vi "Set MenuItem Properties.vi"(0 "NotifyIcon in":refnum<class "NotifyIcon.lvclass">, 5 "MenuItem":refnum<k24>, 9 "MenuItem Properties":T1={"Enabled"=TRUE, "Visible"=TRUE, "DefaultItem"=FALSE, "Checked"=FALSE, "RadioCheck"=FALSE, "Break"=FALSE, "BarBreak"=FALSE, "Text"=""}, 11 "error in (no error)":errorcluster) -> (4 "dub NotifyIcon":refnum<class "NotifyIcon.lvclass">, 6 "MenuItem out":refnum<k24>, 15 "error out":errorcluster)   [LabVIEW 2016, in "NotifyIcon.lvclass"]
doc: "This VI sets the properties for the MenuItem referenced by the <b>MenuItem</b> input.\n\n\nStinus Olsen\nCIM Industrial Systems A/S\n22. Feb. 2011 15:06\nmailto: seo@cim.as"
uses:
  NotifyIcon.lvclass
  System.Windows.Forms
  Controls/MenuItem Properties.ctl
panel:
  # "This VI belongs to the NotifyIcon Toolset. \nA toolset that makes it easy to create, control and manipulate a notification icon in the notification area of the Windows taskbar.\nThe toolset requires Microsoft .NET framework 2.0\n\n\nNOTICE -- YOU MUST LEAVE THIS NOTICE IN PLACE.  PER THE TERMS OF THE LICENSE BELOW, YOU MAY SUBLICENSE THIS SOFTWARE \nIN ANY WAY THAT DOES NOT CONFLICT WITH THIS LICENSE.\n\n### BSD License (http://www.opensource.org/licenses/bsd-license.php) Begin ###\n \nCopyright (c) 2011, Stinus Olsen <seo@cim.as>\n\nAll rights reserved.\n\nRedistribution and use in source and binary forms, with or without modification, are permitted provided that the following conditions are met:\n\n    * Redistributions of source code must retain the above copyright notice, this list of conditions and the following disclaimer.\n    * Redistributions in binary form must reproduce the above copyright notice, this list of conditions and the following disclaimer in the \n       documentation and/or other materials provided with the distribution.\n    * Neither the name of CIM Industrial Systems nor the names of its contributors may be used to endorse or promote products derived \n       from this software without specific prior written permission.\n\nTHIS SOFTWARE IS PROVIDED BY THE COPYRIGHT HOLDERS AND CONTRIBUTORS \"AS IS\" AND ANY EXPRESS OR IMPLIED WARRANTIES, \nINCLUDING, BUT NOT LIMITED TO, THE IMPLIED WARRANTIES OF MERCHANTABILITY AND FITNESS FOR A PARTICULAR PURPOSE ARE \nDISCLAIMED. IN NO EVENT SHALL THE COPYRIGHT OWNER OR CONTRIBUTORS BE LIABLE FOR ANY DIRECT, INDIRECT, INCIDENTAL,\n SPECIAL, EXEMPLARY, OR CONSEQUENTIAL DAMAGES (INCLUDING, BUT NOT LIMITED TO, PROCUREMENT OF SUBSTITUTE GOODS OR \nSERVICES; LOSS OF USE, DATA, OR PROFITS; OR BUSINESS INTERRUPTION) HOWEVER CAUSED AND ON ANY THEORY OF LIABILITY, \nWHETHER IN CONTRACT, STRICT LIABILITY, OR TORT (INCLUDING NEGLIGENCE OR OTHERWISE) ARISING IN ANY WAY OUT OF THE USE \nOF THIS SOFTWARE, EVEN IF ADVISED OF THE POSSIBILITY OF SUCH DAMAGE.\n\n### BSD License End ###"
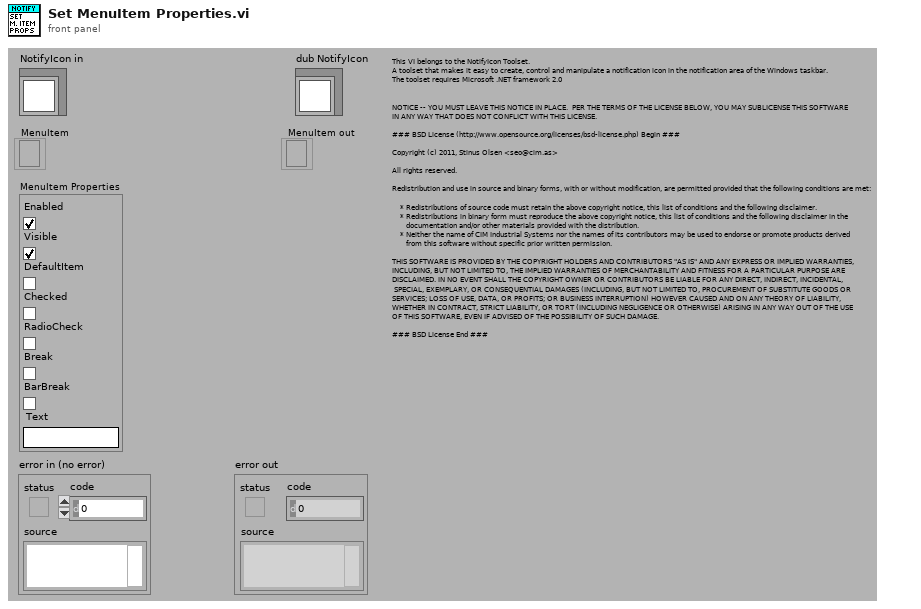
[diagram p1: front panel]
types:
  T1 = typedef "NotifyIcon.lvclass/MenuItem Properties.ctl" = cluster{"Enabled":bool, "Visible":bool, "DefaultItem":bool, "Checked":bool, "RadioCheck":bool, "Break":bool, "BarBreak":bool, "Text":string}
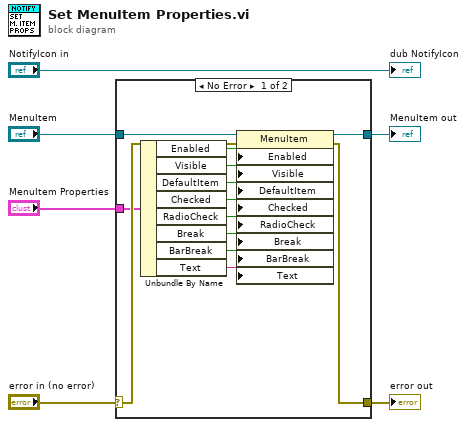
[diagram p0: block diagram]
diagram:
  n1 = case shown="No Error" "error in (no error)" {
    selector: "error in (no error)" -> [w18 w21]
    tunnel: [w17 w21] -> w5
    tunnel: "MenuItem" -> [w19 w20]
    tunnel: [w16 w20] -> w2
    tunnel: "MenuItem Properties" -> [w15 _]
    frame No Error {
      n2 = Unbundle By Name(w15) -> ("Enabled"=w14:bool, "Visible"=w13:bool, "DefaultItem"=w12:bool, "Checked"=w11:bool, "RadioCheck"=w10:bool, "Break"=w9:bool, "BarBreak"=w8:bool, "Text"=w7:string)
      n3 = property class="MenuItem"(reference=w19, error in=w18, "Enabled"=w14, "Visible"=w13, "DefaultItem"=w12, "Checked"=w11, "RadioCheck"=w10, "Break"=w9, "BarBreak"=w8, "Text"=w7) -> (reference out=w16:refnum<k24>, error out=w17:errorcluster)
    }
    frame Error {
    }
  }
  "error out" <- w5
  "MenuItem out" <- w2
  "dub NotifyIcon" <- "NotifyIcon in"
